vi "Pattern Script Generator Test.vi"() -> ()   [LabVIEW 2018]
uses:
  Ctls/Protocol Type.ctl
  Interfaces/File Parser Interface.lvlibp/Interfaces/File Parser Interface/File Parser Interface.lvclass
  Interfaces/Protocol Interface.lvlibp/Interfaces/Protocol Interface/Protocol Interface.lvclass
panel:
  in  "Period(ms)":dbl=0.1 format="%#_13g"
  in  "Wait(ms)":dbl=1.0 format="%#_13g"
  in  "NumofCycleRd":u32=1
  out "Pattern Script out":string
  in  "Protocol Type":T1
  out "error out":errorcluster
  in  "Config File":path
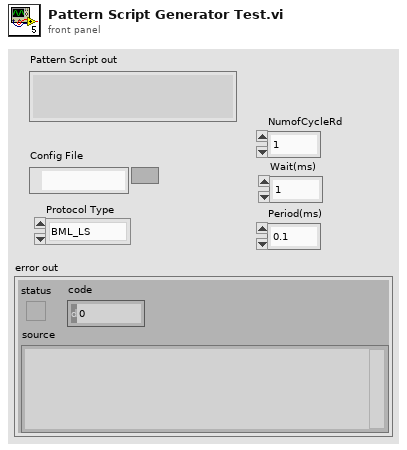
[diagram p1: front panel]
types:
  T1 = typedef "Protocol Type.ctl" = enum16{"BML_LS", "BML_HS", "SPI_3W", "SPI_4W"}
  T2 = enum16{"open", "replace", "create", "open or create", "replace or create", "replace or create with confirmation"}
  T3 = typedef "File Parser Interface.lvlibp/Protocol Type.ctl" = enum16{"BML_LS", "BML_HS", "SPI_3W", "SPI_4W"}
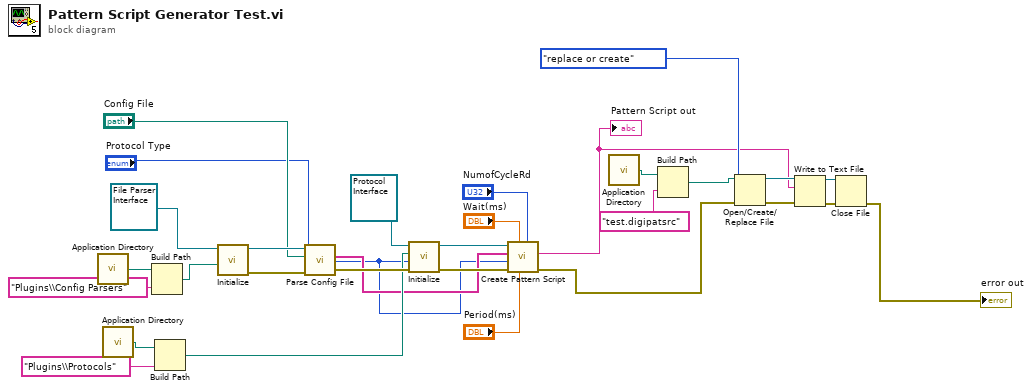
[diagram p0: block diagram]
diagram:
  n1 = call <vilib>:"Application Directory.vi"() -> ("Application Directory"=w31:path)
  n2 = call <vilib>:"Application Directory.vi"() -> ("Application Directory"=w21:path)
  n3 = Build Path(base path=w31, name or relative path="Plugins\\Config Parsers") -> (appended path=w29:path)
  n4 = Build Path(base path=w21, name or relative path="Plugins\\Protocols") -> (appended path=w19:path)
  n5 = call-dynamic "Initialize.vi"("Plugin Folder"=w29, "File Parser Interface in"=refnum<class "File Parser Interface.lvclass"> refnum ("File Parser Interface.lvlibp:File Parser Interface.lvclass")) -> ("error out"=w26:errorcluster, "File Parser Interface out"=w28:refnum<class "File Parser Interface.lvclass">)  [unwired: 8 in]
  n6 = call "Parse Config File.vi"("error in (no error)"=w26, "Protocol Type in"="Protocol Type", "Config File"="Config File", "File Parser Interface in"=w28) -> ("error out"=w22:errorcluster, "Protocol Type out"=w12:T3, "Config Array"=w16:string[])  [unwired: 4 in, 1 out]
  n7 = call "Initialize.vi"("error in (no error)"=w22, "Protocol Type"=w12, "Folder Path"=w19, "Protocol Interface in"=refnum<class "Protocol Interface.lvclass"> refnum) -> ("error out"=w17:errorcluster, "Protocol Interface out"=w18:refnum<class "Protocol Interface.lvclass">)  [unwired: 6 in]
  n8 = call "Create Pattern Script.vi"("NumofCycleRd"="NumofCycleRd", "Period(ms)"="Period(ms)", "Wait(ms)"="Wait(ms)", "error in (no error)"=w17, "Protocol Type"=w12, "Config Array"=w16, "Protocol Interface in"=w18) -> ("error out"=w2:errorcluster, "Pattern Script out"=w1:string)  [unwired: 2 in, 1 out]
  "Pattern Script out" <- w1
  n9 = call <vilib>:"Application Directory.vi"() -> ("Application Directory"=w11:path)
  n10 = Build Path(base path=w11, name or relative path="test.digipatsrc") -> (appended path=w4:path)
  n11 = Open/Create/Replace File(file path (use dialog)=w4, error in=w2, operation (0:open)=T2."replace or create") -> (refnum out=w6:refnum<file>, error out=w5:errorcluster)  [unwired: 3 in, 1 out]
  n12 = Write to Text File(file (use dialog)=w6, text=w1, error in=w5) -> (refnum out=w9:refnum<file>, error out=w8:errorcluster)  [unwired: 1 in, 1 out]
  n13 = Close File(refnum=w9, error in=w8) -> (error out=→"error out":errorcluster)  [unwired: 1 out]
